vi "Proj3_Wireless_DTMF_Shell (Simulate).vi"() -> ()   [LabVIEW 2011]
panel:
  in  "Ringtone Path":path=path "C:/Users/Sungeun/Dropbox/Lab/DTMF/VI Source/Project 3/ringtone/Nokia_Original.wav"
  in  "My Phone Number":string
  out "Received Quantized DTMF Signal":dbl[](graph)
  out "Received Digits":string
  out "Transmitted DTMF Signal":dbl[][](graph)
  in  "Tab Control":enum32{"DTMF", "Quantization"}(tab)
  in  "Dial Tone":bool
  in  "Phone # String":string
  in  "Ring Tone":bool
  in  "Gray Bit Encoding":bool
  in  "Quantization Level":u16(ring)=4 items=["2"=2, "4"=4, "8"=8, "16"=16]
  # "Project 3: Wireless DTMF Transceiver Shell (Simulate)"
  # "Receiver"
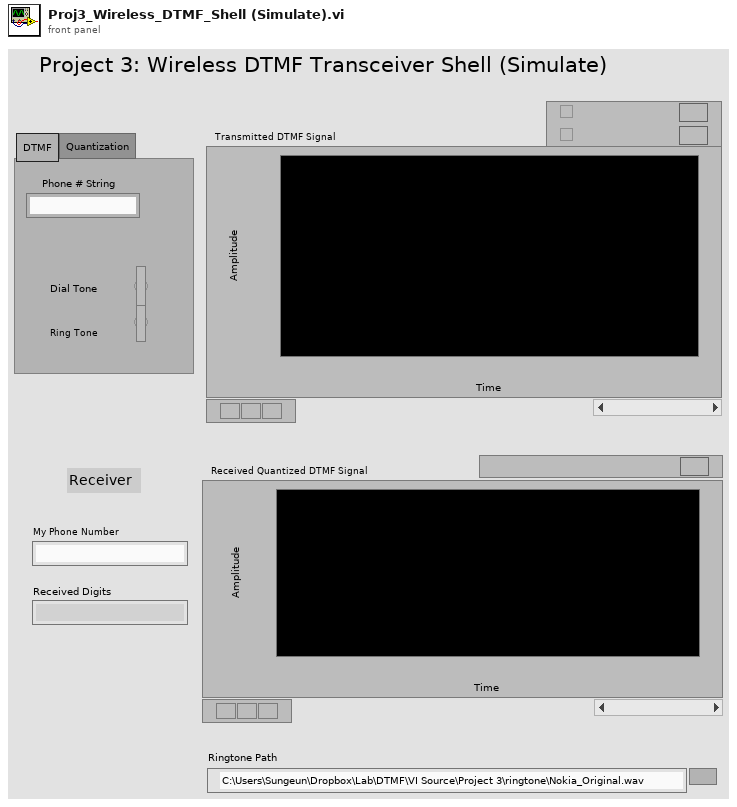
[diagram p1: front panel]
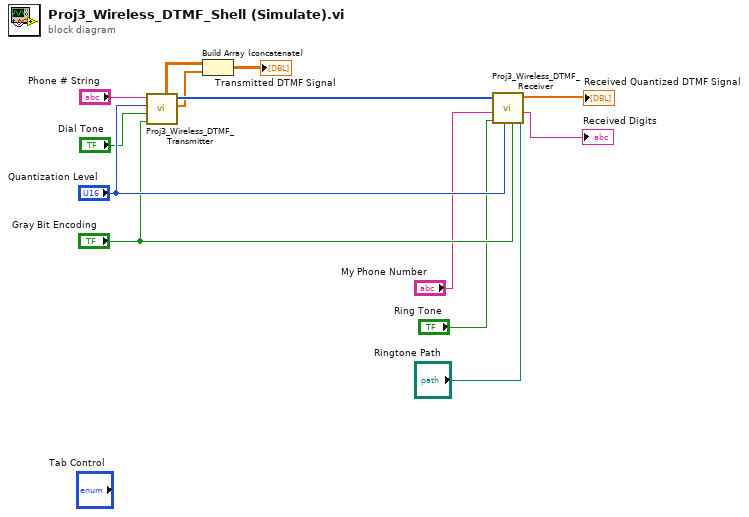
[diagram p0: block diagram]
diagram:
  n1 = call "Proj3_Wireless_DTMF_Transmitter.vi"("Gray Bit Encoding"="Gray Bit Encoding", "Dial Tone"="Dial Tone", "Quantization Level"="Quantization Level", "Phone # String"="Phone # String") -> ("quants"=w3:dbl[], "TXbitStream"=w13:i8[], "TX DTMF Signal"=w4:dbl[][])  [unwired: 1 in, 2 out]
  n2 = Build Array (concatenate)(w4, w3) -> (→"Transmitted DTMF Signal":dbl[][])
  n3 = call "Proj3_Wireless_DTMF_Receiver.vi"("Ringtone Path"="Ringtone Path", "Gray Bit Encoding"="Gray Bit Encoding", "Quantization Level"="Quantization Level", "Ringtone"="Ring Tone", "My Phone Number"="My Phone Number", "RXbitStream"=w13) -> ("Received Digits"=→"Received Digits":string, "dequants"=→"Received Quantized DTMF Signal":dbl[])  [unwired: 4 in]
